vi "niScope Close.vi"(0 "instrument handle":refnum<k15>, 11 "error in":errorcluster) -> (15 "error out":errorcluster)   [LabVIEW 2013]
doc: "Performs the following actions:\n\n-Closes the instrument I/O session.\n\n-Destroys the IVI session and all of its properties.\n\n-Deallocates any memory resources used by the IVI session.\n\nCall this VI when you are finished using an instrument driver session."
uses:
  niScope_32.dll
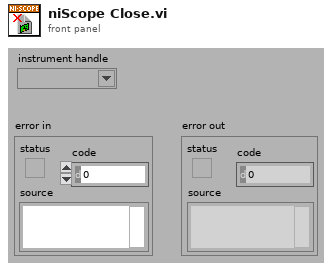
[diagram p1: front panel]
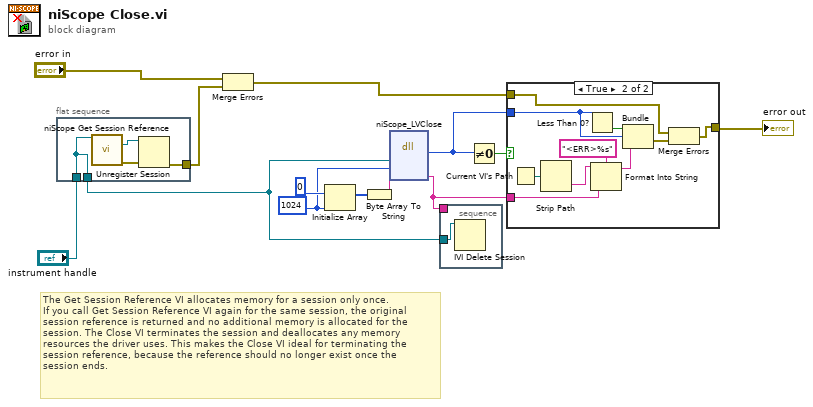
[diagram p0: block diagram]
diagram:
  w6 = 1024
  # "The Get Session Reference VI allocates memory for a session only once.  \nIf you call Get Session Reference VI again for the same session, the original \nsession reference is returned and no additional memory is allocated for the \nsession. The Close VI terminates the session and deallocates any memory \nresources the driver uses. This makes the Close VI ideal for terminating the \nsession reference, because the reference should no longer exist once the \nsession ends."
  n1 = flat-sequence {
    tunnel: "instrument handle" -> [w14]
    tunnel: [w17] -> w10
    tunnel: [w14] -> w1
    frame #0 {
      n2 = call "niScope Get Session Reference.vi"("instrument handle"=w14) -> ("session reference"=w15:refnum<k20>, "error out"=w16:errorcluster)  [unwired: 12 in, 1 out]
      n3 = Unregister Session(8:w16, 11:w15) -> (0:w17:errorcluster)
    }
  }
  n4 = Merge Errors("error in", w10) -> (w12:errorcluster)
  n5 = Initialize Array(0, w6) -> (w7:i32[])
  n6 = Byte Array To String(unsigned byte array=w7) -> (string=w5:string)
  n7 = dll-call lib="niScope_*.*" fn="niScope_LVClose"("instrument handle"=w1, "buffer size"=w6, "error buffer"=w5) -> ("status"=w2:i32, "error buffer"=w4:string)  [unwired: 5 in, 2 out]
  n8 = stacked-sequence {
    tunnel: w1 -> [w18]
    tunnel: w4 -> [_]
    frame #0 {
      n9 = IVI Delete Session(11:w18) -> ()
    }
  }
  n10 = Not Equal To 0?(x=w2) -> (x != 0?=w3:bool)
  n11 = case shown="True" w3 {
    tunnel: w2 -> [_ w24]
    tunnel: w4 -> [_ w27]
    tunnel: [w19 w20] -> w13
    tunnel: w12 -> [w19 w22]
    frame False {
    }
    frame True {
      n12 = Current VI's Path() -> (path=w29:path)
      n13 = Strip Path(path=w29) -> (name=w28:string)  [unwired: 1 out]
      n14 = Less Than 0?(x=w24) -> (x < 0?=w23:bool)
      n15 = Format Into String(format string="<ERR>%s" ("Format String"), initial string=w28, w27) -> (resulting string=w25:string)  [unwired: 1 in, 1 out]
      n16 = Bundle(w23, "status"=w24, w25) -> (w21:cluster{bool, "status":i32, string})  [unwired: 1 in]
      n17 = Merge Errors(w22, w21) -> (w20:errorcluster)
    }
  }
  "error out" <- w13
